vi "Untitled 1.vi"() -> ()   [LabVIEW 2019, in "Instrument.LN2.lvclass"]
uses:
  Instrument.LN2.lvclass
  <vilib>/regexp/Match Regular Expression.xnode
panel:
  out "before match":string
  out "output 2":dbl
  out "after match":string
  out "output 1":dbl
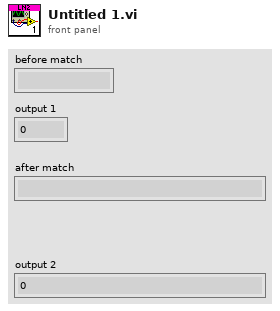
[diagram p1: front panel]
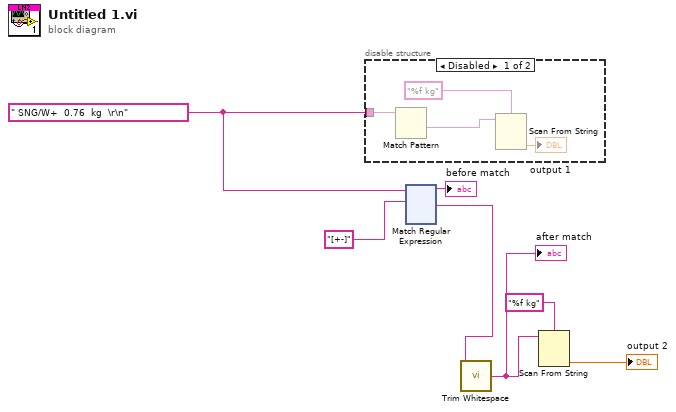
[diagram p0: block diagram]
diagram:
  w7 = " SNG/W+  0.76  kg  \r\n" ("read buffer")
  n1 = disable-structure shown="Disabled" {
    disable-tunnel: w7 -> [w8 _]
    frame Disabled {
      n2 = Match Pattern(string=w8) -> (after substring=w9:string)  [unwired: 2 in, 3 out]
      n3 = Scan From String(format string="%f kg", input string=w9) -> (output 1=→"output 1":dbl)  [unwired: 3 in, 3 out]
    }
    frame Enabled {
    }
  }
  n4 = xnode "Match Regular Expression"("input string"=w7, "regular expression"="[+-]" ("format string")) -> ("before match"=→"before match":string, "after match"=w2:string)  [unwired: 4 in, 3 out]
  n5 = call <vilib>:"Trim Whitespace.vi"("string"=w2) -> ("trimmed string"=w1:string)  [unwired: 1 in]
  "after match" <- w1
  n6 = Scan From String(format string="%f kg", input string=w1) -> (output 1=→"output 2":dbl)  [unwired: 3 in, 3 out]
